vi "tEST FGV-BroadcastRegistry.vi"() -> ()   [LabVIEW 2014]
uses:
  user.lib/_NEVSTOP/JKI State Machine ++/_Support/FGV-BroadcastRegistry/Oper-BroadcastRegistry.ctl
  user.lib/_NEVSTOP/JKI State Machine ++/JKI-State-Machine-Plus.lvlib
panel:
  out "ActingMsg out 4":string="STATUS"
  out "ActingMsg out 3":string="STATUS"
  out "ActingMsg out 2":string="STATUS"
  out "ActingMsg out":string="STATUS"
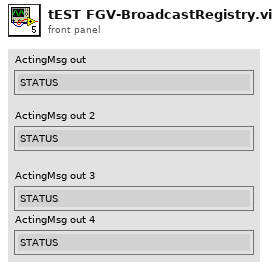
[diagram p1: front panel]
types:
  T1 = typedef "JKI-State-Machine-Plus.lvlib/Oper-BroadcastRegistry.ctl" = enum16{"Delete Source Module", "Delete Dest Module", "Remove Module", "Register", "Unregister", "Check"}
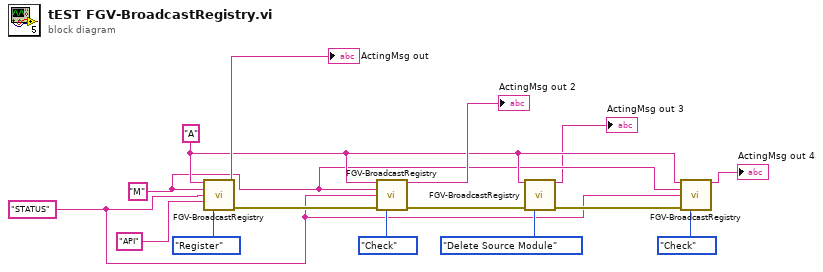
[diagram p0: block diagram]
diagram:
  w3 = "STATUS" ("Message")
  w4 = "M" ("Dest")
  w5 = "A" ("Source")
  n1 = call "FGV-BroadcastRegistry.vi"("Source"=w5, "Dest"=w4, "Message"=w3, "ActingMsg In"="API", "Operation"=Oper-BroadcastRegistry."Register") -> ("ActingMsg out"=→"ActingMsg out":string, "Error out"=w12:errorcluster)  [unwired: 8 in, 1 out]
  n2 = call "FGV-BroadcastRegistry.vi"("Source"=w5, "Dest"=w4, "Message"=w3, "Error in"=w12, "Operation"=Oper-BroadcastRegistry."Check") -> ("ActingMsg out"=→"ActingMsg out 2":string, "Error out"=w9:errorcluster)  [unwired: 8 in, 1 out]
  n3 = call "FGV-BroadcastRegistry.vi"("Source"=w5, "Error in"=w9, "Operation"=Oper-BroadcastRegistry."Delete Source Module") -> ("ActingMsg out"=→"ActingMsg out 3":string, "Error out"=w6:errorcluster)  [unwired: 10 in, 1 out]
  n4 = call "FGV-BroadcastRegistry.vi"("Source"=w5, "Dest"=w4, "Message"=w3, "Error in"=w6, "Operation"=Oper-BroadcastRegistry."Check") -> ("ActingMsg out"=→"ActingMsg out 4":string)  [unwired: 8 in, 2 out]
